vi "流程写入.vi"(11 "添加的路径":path) -> ()   [LabVIEW 2016, in "斯坦道总磷.lvlib"]
uses:
  <vilib>/Utility/miscctls.llb/LVPointTypeDef.ctl
panel:
  in  "关闭":bool
  out "字符串":string
  in  "加标回收":bool
  in  "标样核查":bool
  in  "跨度核查":bool
  in  "零点核查":bool
  in  "水样测量":bool=TRUE
  in  "写入":bool
  in  "参数下拉列表":enum16{"COD", "氨氮", "总氮", "总磷"}(ring)
  in  "量程下拉列表":enum16{"低量程", "高量程"}(ring)
  # "请选择要写入的流程"
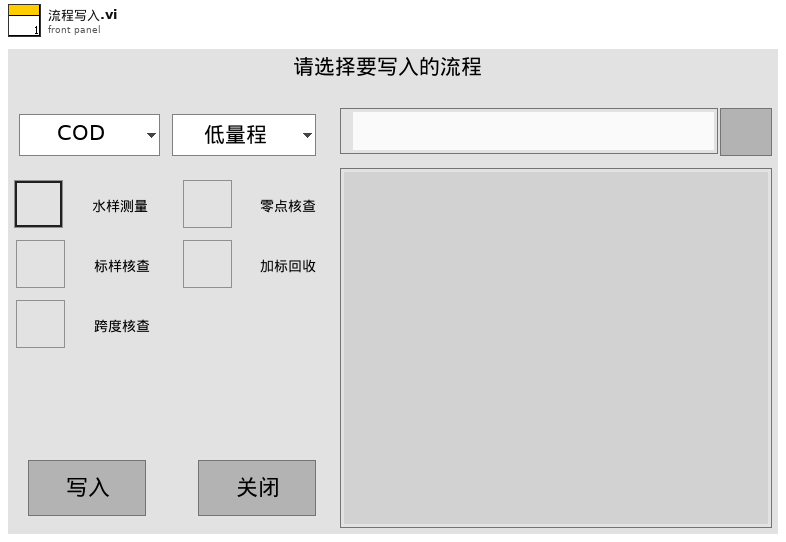
[diagram p1: front panel]
types:
  T1 = typedef "LVPointTypeDef.ctl" = cluster{"Horizontal":i16, "Vertical":i16}
  T2 = cluster{"COD":bool, "氨氮":bool, "总氮":bool, "总磷":bool}
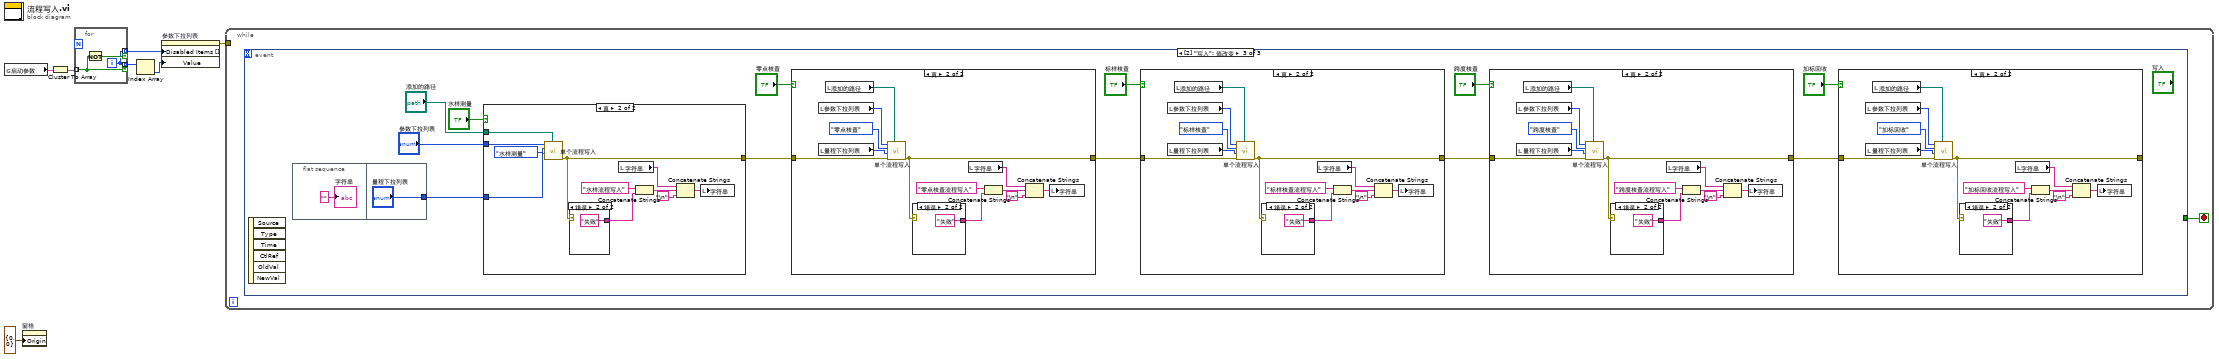
[diagram p0: block diagram]
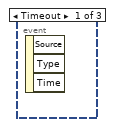
[diagram p2: hidden frame]
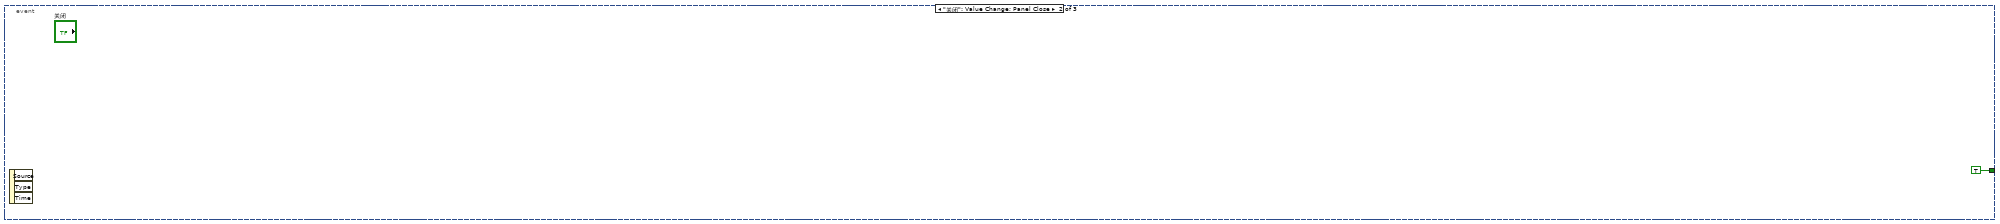
[diagram p3: hidden frame]
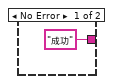
[diagram p5: hidden frame]
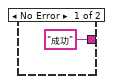
[diagram p7: hidden frame]
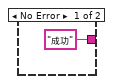
[diagram p9: hidden frame]
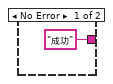
[diagram p11: hidden frame]
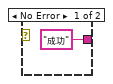
[diagram p13: hidden frame]
diagram:
  n1 = global read "总磷总氮断电保存全局变量.vi" "启动参数"() -> (w4:T2)
  n2 = property on="窗格" class="Pane"("Origin"=T1 {"Horizontal"=0, "Vertical"=0} ("原点")) -> ()  [unwired: 2 in, 2 out]
  n3 = Cluster To Array(cluster=w4) -> (array=w5:bool[])
  n4 = for {
    tunnel: w5 -> [w8] mode=indexing
    tunnel: [w9] -> w2 mode=indexing if=w10
    tunnel: [w9] -> w6 mode=indexing if=w8
    i -> [w9]
    n5 = Not(x=w8) -> (.not. x?=w10:bool)
  }
  n6 = Index Array(array=w6) -> (element=w3:i32)  [unwired: 1 in]
  n7 = property on="参数下拉列表" class="Enum (严格)"("Disabled Items []"=w2, "Value"=w3) -> (error out=w1:errorcluster)  [unwired: 2 in, 1 out]
  n8 = while {
    tunnel: w1 -> [_]
    stop <- w11 stop-if-true
    n9 = event shown="[2] \"写入\": 值改变" {
      selector: _ -> [_ _ _]
      dyn-events: _ -> [_ _ _]
      timeout: _ -> [_ _ _]
      tunnel: [_ TRUE _] -> w11
      event Timeout {
        n10 = event-data() -> ()  [unwired: 1 in, 3 out]
      }
      event "关闭": Value Change; Panel Close {
        n11 = event-data() -> ()  [unwired: 1 in, 3 out]
      }
      event "写入": Value Change {
        n12 = event-data() -> ()  [unwired: 1 in, 6 out]
        n13 = flat-sequence {
          tunnel: ["量程下拉列表"] -> w23
          frame #0 {
            "字符串" <- ""
          }
          frame #1 {
          }
        }
        n14 = case shown="真" "水样测量" {
          tunnel: "添加的路径" -> [_ w93]
          tunnel: "参数下拉列表" -> [_ w92]
          tunnel: w23 -> [_ w91]
          tunnel: [_ w89] -> w20
          frame False {
          }
          frame True {
            n15 = call "单个流程写入.vi"("添加的路径"=w93, "量程"=w91, "测量模式"=enum16{"水样测量", "零点核查", "跨度核查", "标样核查", "加标回收"}."水样测量", "测量参数"=w92) -> ("error out"=w89:errorcluster)  [unwired: 6 in, 1 out]
            n16 = case shown="错误" w89 {
              tunnel: ["成功" "失败"] -> w86
              frame No Error {
              }
              frame Error {
              }
            }
            n17 = local read "字符串"() -> (w88:string)
            n18 = Concatenate Strings("水样流程写入", w86) -> (w85:string)
            n19 = Concatenate Strings(w88, w85, "\n") -> (w83:string)
            n20 = local write "字符串"(w83) -> ()
          }
        }
        n21 = case shown="真" "零点核查" {
          tunnel: [_ w79] -> w18
          tunnel: w20 -> [_ w69]
          frame False {
          }
          frame True {
            n22 = local read "参数下拉列表"() -> (w71:enum16{"COD", "氨氮", "总氮", "总磷"})
            n23 = local read "量程下拉列表"() -> (w70:enum16{"低量程", "高量程"})
            n24 = local read "添加的路径"() -> (w72:path)
            n25 = call "单个流程写入.vi"("添加的路径"=w72, "error in (no error)"=w69, "量程"=w70, "测量模式"=enum16{"水样测量", "零点核查", "跨度核查", "标样核查", "加标回收"}."零点核查", "测量参数"=w71) -> ("error out"=w79:errorcluster)  [unwired: 5 in, 1 out]
            n26 = case shown="错误" w79 {
              tunnel: ["成功" "失败"] -> w76
              frame No Error {
              }
              frame Error {
              }
            }
            n27 = local read "字符串"() -> (w78:string)
            n28 = Concatenate Strings("零点核查流程写入", w76) -> (w75:string)
            n29 = Concatenate Strings(w78, w75, "\n") -> (w73:string)
            n30 = local write "字符串"(w73) -> ()
          }
        }
        n31 = case shown="真" "标样核查" {
          tunnel: [_ w65] -> w16
          tunnel: w18 -> [_ w55]
          frame False {
          }
          frame True {
            n32 = local read "参数下拉列表"() -> (w57:enum16{"COD", "氨氮", "总氮", "总磷"})
            n33 = local read "量程下拉列表"() -> (w56:enum16{"低量程", "高量程"})
            n34 = local read "添加的路径"() -> (w58:path)
            n35 = call "单个流程写入.vi"("添加的路径"=w58, "error in (no error)"=w55, "量程"=w56, "测量模式"=enum16{"水样测量", "零点核查", "跨度核查", "标样核查", "加标回收"}."标样核查", "测量参数"=w57) -> ("error out"=w65:errorcluster)  [unwired: 5 in, 1 out]
            n36 = case shown="错误" w65 {
              tunnel: ["成功" "失败"] -> w62
              frame No Error {
              }
              frame Error {
              }
            }
            n37 = local read "字符串"() -> (w64:string)
            n38 = Concatenate Strings("标样核查流程写入", w62) -> (w61:string)
            n39 = Concatenate Strings(w64, w61, "\n") -> (w59:string)
            n40 = local write "字符串"(w59) -> ()
          }
        }
        n41 = case shown="真" "跨度核查" {
          tunnel: [_ w41] -> w13
          tunnel: w16 -> [_ w42]
          frame False {
          }
          frame True {
            n42 = local read "参数下拉列表"() -> (w44:enum16{"COD", "氨氮", "总氮", "总磷"})
            n43 = local read "量程下拉列表"() -> (w43:enum16{"低量程", "高量程"})
            n44 = local read "添加的路径"() -> (w45:path)
            n45 = call "单个流程写入.vi"("添加的路径"=w45, "error in (no error)"=w42, "量程"=w43, "测量模式"=enum16{"水样测量", "零点核查", "跨度核查", "标样核查", "加标回收"}."跨度核查", "测量参数"=w44) -> ("error out"=w41:errorcluster)  [unwired: 5 in, 1 out]
            n46 = case shown="错误" w41 {
              tunnel: ["成功" "失败"] -> w49
              frame No Error {
              }
              frame Error {
              }
            }
            n47 = local read "字符串"() -> (w51:string)
            n48 = Concatenate Strings("跨度核查流程写入", w49) -> (w48:string)
            n49 = Concatenate Strings(w51, w48, "\n") -> (w46:string)
            n50 = local write "字符串"(w46) -> ()
          }
        }
        n51 = case shown="真" "加标回收" {
          tunnel: [_ w37] -> _
          tunnel: w13 -> [_ w27]
          frame False {
          }
          frame True {
            n52 = local read "参数下拉列表"() -> (w29:enum16{"COD", "氨氮", "总氮", "总磷"})
            n53 = local read "量程下拉列表"() -> (w28:enum16{"低量程", "高量程"})
            n54 = local read "添加的路径"() -> (w30:path)
            n55 = call "单个流程写入.vi"("添加的路径"=w30, "error in (no error)"=w27, "量程"=w28, "测量模式"=enum16{"水样测量", "零点核查", "跨度核查", "标样核查", "加标回收"}."加标回收", "测量参数"=w29) -> ("error out"=w37:errorcluster)  [unwired: 5 in, 1 out]
            n56 = case shown="错误" w37 {
              tunnel: ["成功" "失败"] -> w34
              frame No Error {
              }
              frame Error {
              }
            }
            n57 = local read "字符串"() -> (w36:string)
            n58 = Concatenate Strings("加标回收流程写入", w34) -> (w33:string)
            n59 = Concatenate Strings(w36, w33, "\n") -> (w31:string)
            n60 = local write "字符串"(w31) -> ()
          }
        }
      }
    }
  }
